vi "Signals to JSON 3.vi"() -> ()   [LabVIEW 2021]
uses:
  5eec69ea-4072-4200-a2f8-4861d0f2fd1f.vi
  <vilib>/JDP Science/JSONtext/Variant to JSON Text.vi
  <vilib>/JDP Science/JSONtext/LVClass Serializer/JSONtext LVClass Serializer.lvclass
panel:
  out "JSON string":string
  in  "Signal Sessions":T1
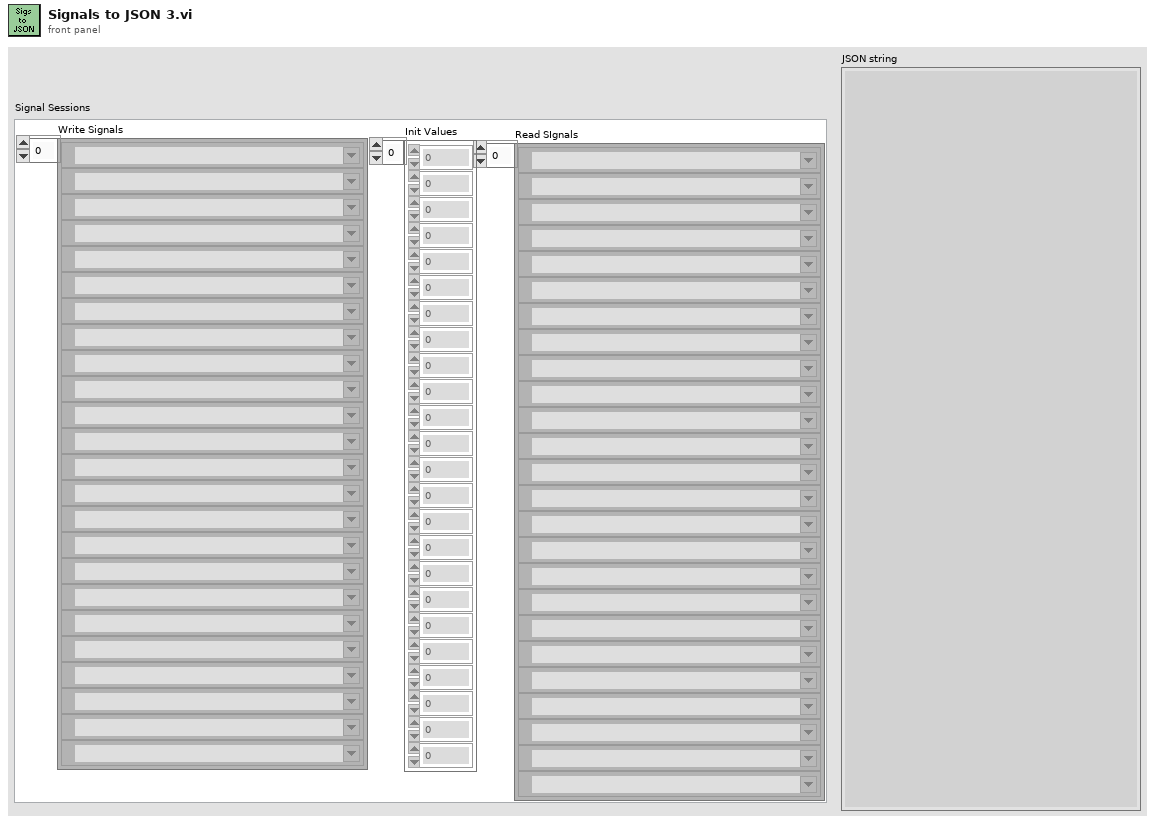
[diagram p1: front panel]
types:
  T1 = cluster{"Read SIgnals":refnum<k21>[], "Write Signals":refnum<k21>[], "Init Values":i32[]}
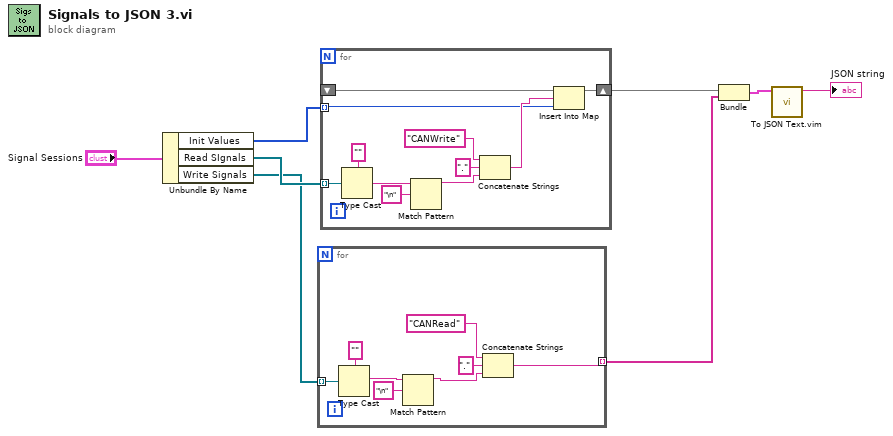
[diagram p0: block diagram]
diagram:
  n1 = Unbundle By Name("Signal Sessions") -> ("Init Values"=w5:i32[], "Read SIgnals"=w7:refnum<k21>[], "Write Signals"=w6:refnum<k21>[])
  n2 = for {
    tunnel: w6 -> [w15] mode=indexing
    tunnel: [w9] -> w3 mode=indexing
    n3 = Type Cast(type="", x=w15) -> (*(type *) &x=w11:string)
    n4 = Match Pattern(string=w11, regular expression="\n") -> (before substring=w10:string)  [unwired: 1 in, 3 out]
    n5 = Concatenate Strings("CANRead" ("type"), "." ("string"), w10) -> (w9:string)
  }
  n6 = for {
    tunnel: w7 -> [w26] mode=indexing
    tunnel: w5 -> [w19] mode=indexing
    shift-right: [w18] -> w2
    shift-left: _ -> [w17]
    n7 = Type Cast(type="", x=w26) -> (*(type *) &x=w23:string)
    n8 = Match Pattern(string=w23, regular expression="\n") -> (before substring=w21:string)  [unwired: 1 in, 3 out]
    n9 = Concatenate Strings("CANWrite" ("type"), "." ("string"), w21) -> (w20:string)
    n10 = Insert Into Map(map in=w17, key=w20, value=w19) -> (map out=w18:map{string, i32})  [unwired: 2 out]
  }
  n11 = Bundle(w2, w3) -> (w1:cluster{map{string, i32}, string[]})  [unwired: 1 in]
  n12 = call "To JSON Text.vim"("Anything"=w1) -> ("<JSON>"=→"JSON string":string)  [unwired: 9 in, 1 out]
